vi "Autonomous Independent.vi"() -> ()   [LabVIEW 2015]
doc: "This VI is called when autonomous begins, and will automatically be terminated when autonomous ends. You can carry out timed or sensor driven robot movement independently without needing to return to the caller."
uses:
  <vilib>/Rock Robotics/WPI/Utilities/WPI_GetSetVariantRefNum.vi
  <vilib>/Rock Robotics/WPI/RobotDrive/WPI_RobotDriveArcadeDrive_Standard(NoSaturation).vi
panel:
  in  "Array of robot movements":T1(array[cluster]) {"Y Joystick Value" scale=1.0..-1.0; "X Joystick Value" scale=-1.0..1.0}
  out "Current Movement, for debugging":T2 {"Y Joystick Value" scale=1.0..-1.0; "X Joystick Value" scale=-1.0..1.0}
  # "Be sure to right-click and choose Data Operations>>Make Current Value default if you want to save the array values with the VI"
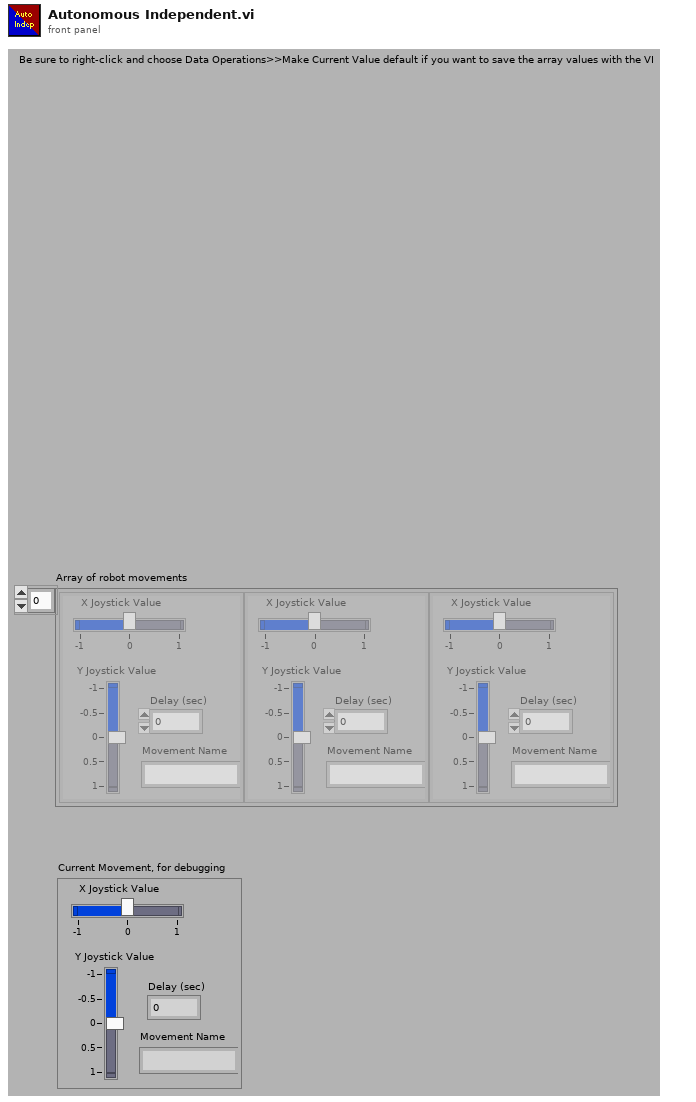
[diagram p1: front panel]
types:
  T1 = cluster{"X Joystick Value":dbl, "Y Joystick Value":dbl, "Delay (sec)":dbl, "Movement Name":string}[]
  T2 = cluster{"X Joystick Value":dbl, "Y Joystick Value":dbl, "Delay (sec)":dbl, "Movement Name":string}
  T3 = typedef "WPI_RobotDriveDevRef.ctl" = cluster{"DevStatus":errorcluster, "Motors[]":T4[], "Square Inputs":bool, "Max Output":dbl}
  T4 = typedef "WPI_MotorControlDeviceRef.ctl" = cluster{"DeviceStatus":errorcluster, "Type":T5, "PWM":cluster{"PWM Channel":T6, "DeadBand":T7}, "CAN":cluster{"Device Number":u8, "Control Mode":T8, "Semaphore":T9, "Max Vout":dbl, "TalonSRX Control Mode":T10}, "Invert":bool}
  T5 = typedef "WPI_MotorControlType.ctl" = enum16{"PWM", "CAN", "CANTalonSRX"}
  T6 = typedef "FPGA_DIOPWMChannel.ctl" = enum8{"PWM 0", "PWM 1", "PWM 2", "PWM 3", "PWM 4", "PWM 5", "PWM 6", "PWM 7", "PWM 8", "PWM 9", "PWM MXP 0", "PWM MXP 1", "PWM MXP 2", "PWM MXP 3", "PWM MXP 4", "PWM MXP 5", "PWM MXP 6", "PWM MXP 7", "PWM MXP 8", "PWM MXP 9", "Invalid"}
  T7 = typedef "WPI_PWMDeadband.ctl" = cluster{"Name":string, "maxPositivePwm":i32, "minPositivePwm":i32, "centerPwm":i32, "maxNegativePwm":i32, "minNegativePwm":i32, "angularRange":u16}
  T8 = typedef "WPI_CANJaguar_ControlMode.ctl" = enum8{"Percent VBus", "Current", "Speed", "Position", "Voltage"}
  T9 = typedef "Semaphore RefNum" = refnum<k1>
  T10 = typedef "WPI_CANTalonSRX_APIControlMode.ctl" = enum8{"Percent VBus", "Speed", "Position", "Slave", "Unchanged / Invalid", "Voltage Compensation", "Current", "Motion Profile"}
  T11 = typedef "WPI_AOChannelDevRef.ctl" = cluster{"DevStatus":errorcluster, "AO Channel":T12}
  T12 = typedef "WPI_AnalogOutputChannel.ctl" = enum8{"AO MXP 0", "AO MXP 1", "Invalid"}
  T13 = typedef "WPI_JoystickDevRef.ctl" = cluster{"Device":T14}
  T14 = typedef "WPI_JoystickDeviceEnum.ctl" = enum16{"USB 0", "USB 1", "USB 2", "USB 3", "USB 4", "USB 5"}
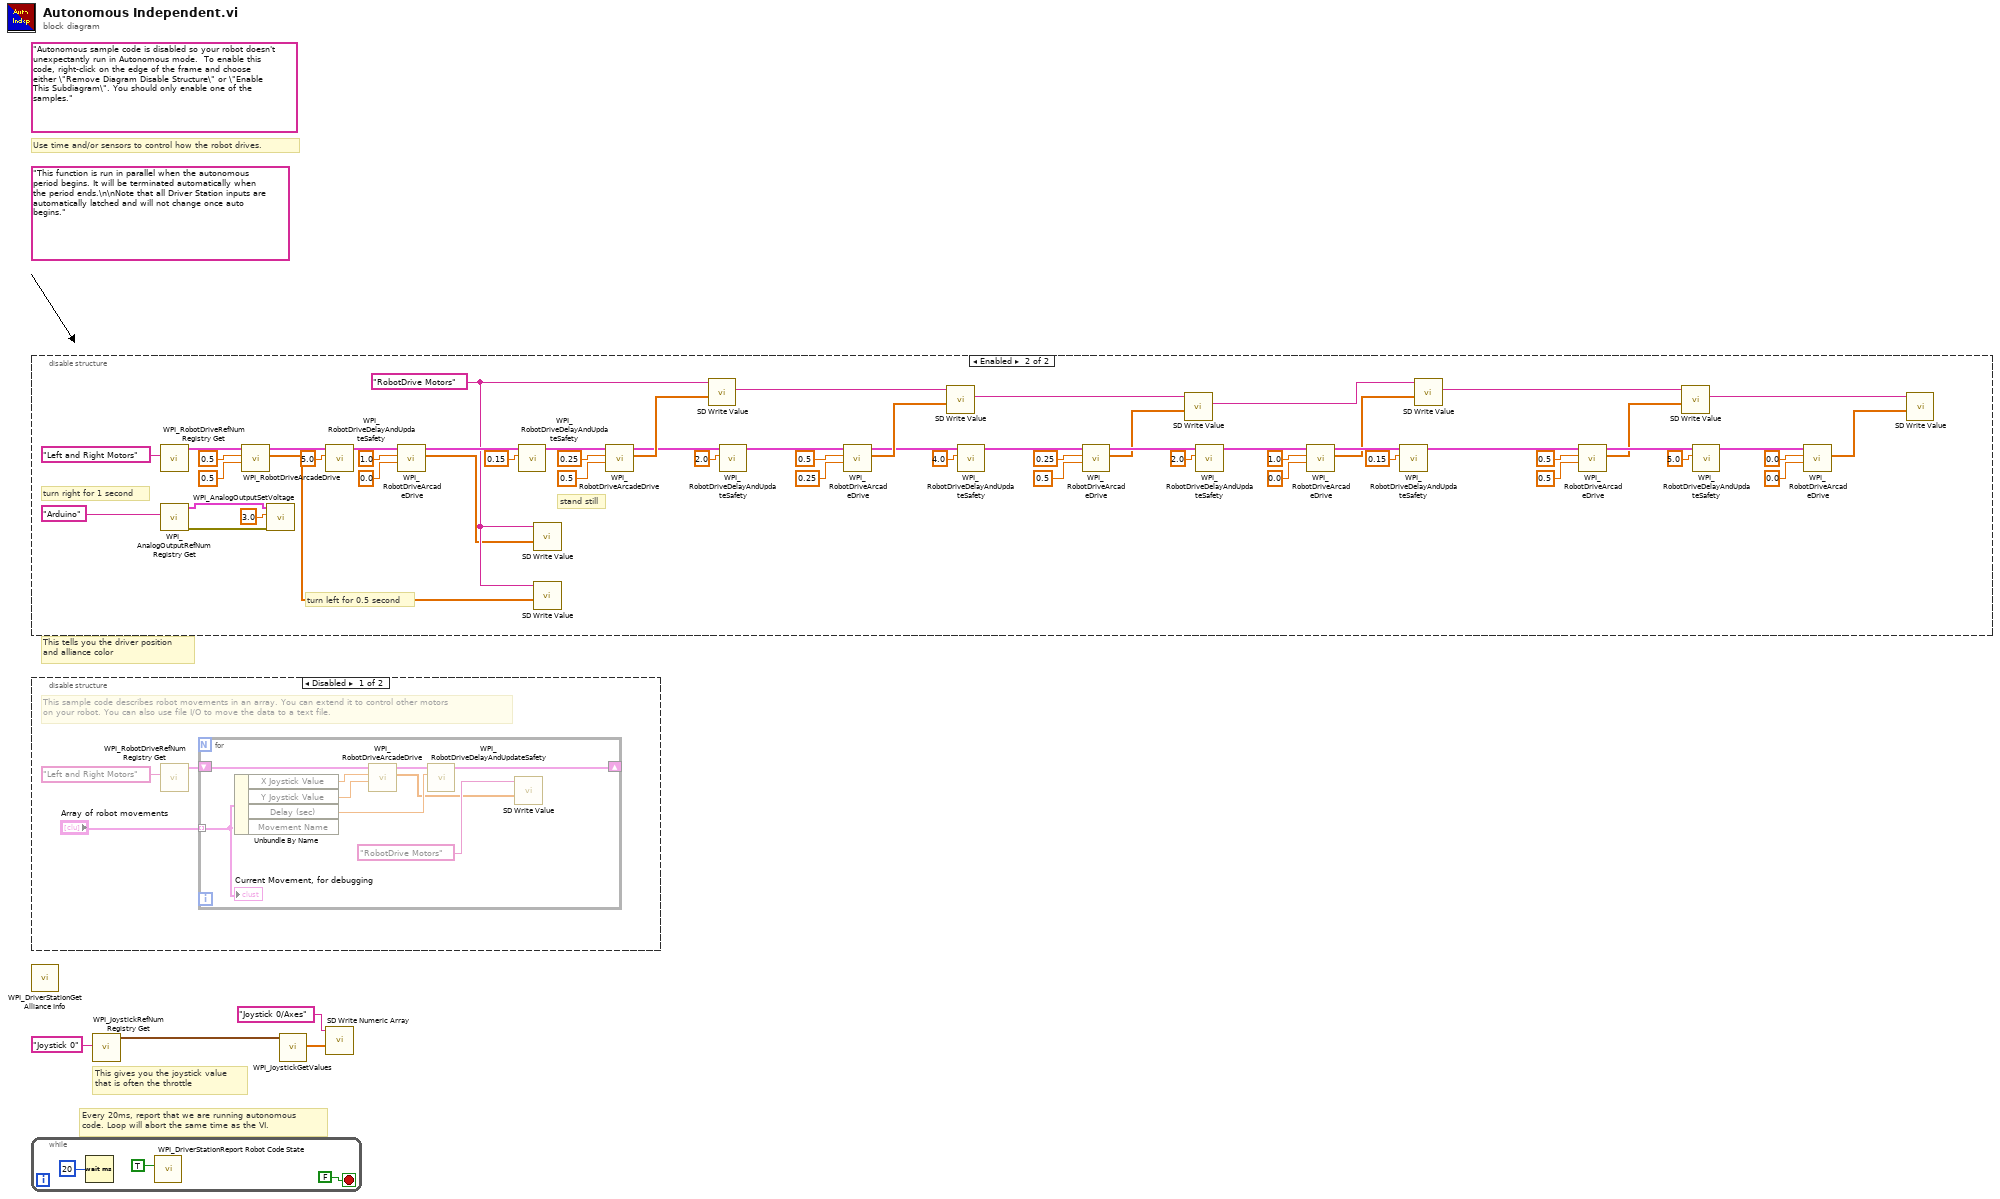
[diagram p0: block diagram]
diagram:
  (unwired) "Autonomous sample code is disabled so your robot doesn't unexpectantly run in Autonomous mode.  To enable this code, right-click on the edge of the frame and choose either \"Remove Diagram Disable Structure\" or \"Enable This Subdiagram\". You should only enable one of the samples."
  (unwired) "This function is run in parallel when the autonomous period begins. It will be terminated automatically when the period ends.\n\nNote that all Driver Station inputs are automatically latched and will not change once auto begins."
  # "Every 20ms, report that we are running autonomous\ncode. Loop will abort the same time as the VI."
  # "This gives you the joystick value\nthat is often the throttle"
  # "Use time and/or sensors to control how the robot drives."
  # "This tells you the driver position\nand alliance color"
  n1 = disable-structure shown="Enabled" {
    frame Disabled {
      # "This is some simple sample code to drive your robot curving one direction and then the other."
    }
    frame Enabled {
      w48 = "RobotDrive Motors" ("Name")
      # "stand still"
      # "turn left for 0.5 second"
      # "turn right for 1 second"
      n2 = call <vilib>:"WPI_RobotDriveRefNum Registry Get.vi"("refnum name"="Left and Right Motors") -> ("RobotDriveDevRef"=w5:T3)  [unwired: 1 in, 9 out]
      n3 = call <vilib>:"WPI_AnalogOutputRefNum Registry Get.vi"("refnum name"="Arduino") -> ("error out"=w8:errorcluster, "AODeviceRef"=w9:T11)  [unwired: 9 in]
      n4 = call-poly <vilib>:"WPI_RobotDriveArcadeDrive.vi"("Y axis value"=0.5 ("X axis value"), "X axis value"=0.5, "RobotDriveDevRef"=w5) -> ("Motor Values"=w47:dbl[], "RobotDriveDevRef"=w55:T3)  [unwired: 1 in, 6 out]
      n5 = call <vilib>:"WPI_AnalogOutputSetVoltage.vi"("error in (no error)"=w8, "Voltage"=3.0, "AODeviceRef"=w9) -> ()  [unwired: 7 in, 2 out]
      n6 = call <vilib>:"WPI_RobotDriveDelayAndUpdateSafety.vi"("Delay (s)"=5.0, "RobotDriveDevRef"=w55) -> ("RobotDriveDevRef 2"=w54:T3)  [unwired: 8 in, 1 out]
      n7 = call-poly <vilib>:"WPI_RobotDriveArcadeDrive.vi"("Y axis value"=0.0 ("X axis value"), "X axis value"=1.0, "RobotDriveDevRef"=w54) -> ("Motor Values"=w46:dbl[], "RobotDriveDevRef"=w53:T3)  [unwired: 1 in, 6 out]
      n8 = call <vilib>:"WPI_RobotDriveDelayAndUpdateSafety.vi"("Delay (s)"=0.15, "RobotDriveDevRef"=w53) -> ("RobotDriveDevRef 2"=w52:T3)  [unwired: 8 in, 1 out]
      n9 = call-poly <vilib>:"SD Write Value.vi"("Numeric Array"=w46, "Name"=w48) -> ()  [unwired: 8 in, 2 out]
      n10 = call-poly <vilib>:"SD Write Value.vi"("Numeric Array"=w47, "Name"=w48) -> ()  [unwired: 8 in, 2 out]
      n11 = call-poly <vilib>:"WPI_RobotDriveArcadeDrive.vi"("Y axis value"=0.5 ("X axis value"), "X axis value"=0.25, "RobotDriveDevRef"=w52) -> ("Motor Values"=w45:dbl[], "RobotDriveDevRef"=w44:T3)  [unwired: 1 in, 6 out]
      n12 = call-poly <vilib>:"SD Write Value.vi"("Numeric Array"=w45, "Name"=w48) -> ("Table Prefix out"=w39:string)  [unwired: 8 in, 1 out]
      n13 = call <vilib>:"WPI_RobotDriveDelayAndUpdateSafety.vi"("Delay (s)"=2.0, "RobotDriveDevRef"=w44) -> ("RobotDriveDevRef 2"=w42:T3)  [unwired: 8 in, 1 out]
      n14 = call-poly <vilib>:"WPI_RobotDriveArcadeDrive.vi"("Y axis value"=0.25, "X axis value"=0.5, "RobotDriveDevRef"=w42) -> ("Motor Values"=w38:dbl[], "RobotDriveDevRef"=w37:T3)  [unwired: 6 in, 1 out]
      n15 = call-poly <vilib>:"SD Write Value.vi"("Numeric Array"=w38, "Name"=w39) -> ("Table Prefix out"=w17:string)  [unwired: 8 in, 1 out]
      n16 = call <vilib>:"WPI_RobotDriveDelayAndUpdateSafety.vi"("Delay (s)"=4.0, "RobotDriveDevRef"=w37) -> ("RobotDriveDevRef 2"=w35:T3)  [unwired: 8 in, 1 out]
      n17 = call-poly <vilib>:"WPI_RobotDriveArcadeDrive.vi"("Y axis value"=0.5, "X axis value"=0.25, "RobotDriveDevRef"=w35) -> ("Motor Values"=w13:dbl[], "RobotDriveDevRef"=w32:T3)  [unwired: 6 in, 1 out]
      n18 = call-poly <vilib>:"SD Write Value.vi"("Numeric Array"=w13, "Name"=w17) -> ("Table Prefix out"=w16:string)  [unwired: 8 in, 1 out]
      n19 = call <vilib>:"WPI_RobotDriveDelayAndUpdateSafety.vi"("Delay (s)"=2.0, "RobotDriveDevRef"=w32) -> ("RobotDriveDevRef 2"=w30:T3)  [unwired: 8 in, 1 out]
      n20 = call-poly <vilib>:"WPI_RobotDriveArcadeDrive.vi"("Y axis value"=0.0, "X axis value"=1.0, "RobotDriveDevRef"=w30) -> ("Motor Values"=w12:dbl[], "RobotDriveDevRef"=w27:T3)  [unwired: 6 in, 1 out]
      n21 = call <vilib>:"WPI_RobotDriveDelayAndUpdateSafety.vi"("Delay (s)"=0.15, "RobotDriveDevRef"=w27) -> ("RobotDriveDevRef 2"=w25:T3)  [unwired: 8 in, 1 out]
      n22 = call-poly <vilib>:"SD Write Value.vi"("Numeric Array"=w12, "Name"=w16) -> ("Table Prefix out"=w15:string)  [unwired: 8 in, 1 out]
      n23 = call-poly <vilib>:"WPI_RobotDriveArcadeDrive.vi"("Y axis value"=0.5, "X axis value"=0.5, "RobotDriveDevRef"=w25) -> ("Motor Values"=w11:dbl[], "RobotDriveDevRef"=w22:T3)  [unwired: 6 in, 1 out]
      n24 = call-poly <vilib>:"SD Write Value.vi"("Numeric Array"=w11, "Name"=w15) -> ("Table Prefix out"=w14:string)  [unwired: 8 in, 1 out]
      n25 = call <vilib>:"WPI_RobotDriveDelayAndUpdateSafety.vi"("Delay (s)"=5.0, "RobotDriveDevRef"=w22) -> ("RobotDriveDevRef 2"=w20:T3)  [unwired: 8 in, 1 out]
      n26 = call-poly <vilib>:"WPI_RobotDriveArcadeDrive.vi"("Y axis value"=0.0, "X axis value"=0.0, "RobotDriveDevRef"=w20) -> ("Motor Values"=w10:dbl[])  [unwired: 6 in, 2 out]
      n27 = call-poly <vilib>:"SD Write Value.vi"("Numeric Array"=w10, "Name"=w14) -> ()  [unwired: 8 in, 2 out]
    }
  }
  n28 = disable-structure shown="Disabled" {
    frame Disabled {
      # "This sample code describes robot movements in an array. You can extend it to control other motors\non your robot. You can also use file I/O to move the data to a text file."
      n29 = call <vilib>:"WPI_RobotDriveRefNum Registry Get.vi"("refnum name"="Left and Right Motors") -> ("RobotDriveDevRef"=w63:T3)  [unwired: 1 in, 9 out]
      n30 = for {
        shift-right: [w70] -> _
        shift-left: w63 -> [w71]
        tunnel: "Array of robot movements" -> [w66] mode=indexing
        n31 = Unbundle By Name(w66) -> ("X Joystick Value"=w69:dbl, "Y Joystick Value"=w68:dbl, "Delay (sec)"=w67:dbl)  [unwired: 1 out]
        n32 = call-poly <vilib>:"WPI_RobotDriveArcadeDrive.vi"("Y axis value"=w68, "X axis value"=w69, "RobotDriveDevRef"=w71) -> ("Motor Values"=w65:dbl[], "RobotDriveDevRef"=w72:T3)  [unwired: 1 in, 6 out]
        n33 = call <vilib>:"WPI_RobotDriveDelayAndUpdateSafety.vi"("Delay (s)"=w67, "RobotDriveDevRef"=w72) -> ("RobotDriveDevRef 2"=w70:T3)  [unwired: 8 in, 1 out]
        n34 = call-poly <vilib>:"SD Write Value.vi"("Numeric Array"=w65, "Name"="RobotDrive Motors") -> ()  [unwired: 8 in, 2 out]
        "Current Movement, for debugging" <- w66
      }
    }
    frame Enabled {
    }
  }
  n35 = call <vilib>:"WPI_DriverStationGet Alliance Info.vi"() -> ()  [unwired: 12 out]
  n36 = while {
    stop <- FALSE stop-if-true
    n37 = Wait (ms)(milliseconds to wait=u32 20) -> ()  [unwired: 1 out]
    n38 = call <vilib>:"WPI_DriverStationReport Robot Code State.vi"("Autonomous"=TRUE) -> ()  [unwired: 10 in, 1 out]
  }
  n39 = call <vilib>:"WPI_JoystickRefNum Registry Get.vi"("refnum name"="Joystick 0") -> ("JoystickDevRef"=w3:T13)  [unwired: 1 in, 9 out]
  n40 = call <vilib>:"WPI_JoystickGetValues.vi"("JoystickDevRef"=w3) -> ("Axes"=w1:dbl[])  [unwired: 6 in, 4 out]
  n41 = call <vilib>:"SD Write Numeric Array.vi"("Numeric Array"=w1, "Name"="Joystick 0/Axes") -> ()  [unwired: 8 in, 2 out]
